vi "Poly_Micro_Delay.vi"   [LabVIEW 2012]
doc: "Causes the script to wait the specified number of micro-seconds before continuing to execute."
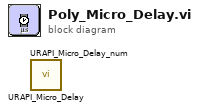
[diagram p0: block diagram]
diagram:
  n1 = call <userlib>:"URAPI_Micro_Delay.vi"() -> ()  [unwired: 5 in, 1 out]
  n2 = call <userlib>:"URAPI_Micro_Delay_num.vi"() -> ()  [unwired: 5 in, 1 out]
